vi "state-counter.vi"(10 "state-idx":u8) -> ()   [LabVIEW 2017]
uses:
  <vilib>/rvi/Emulation/niFpgaEmulationIsFPGAContextNoSignature.vi
  <vilib>/rvi/DataTransferAndStorage/Container/Common/niFpgaContainerGetUniqueNameForEmu.vi
  <vilib>/rvi/Memory/Memory_Emulation/niFpgaMemoryEmulationCacheClearOnFirstRun.vi
  <vilib>/rvi/Memory/Memory_Emulation/nirvimemoryEmulationManagerCache_MakeExclusive.vi
  <vilib>/rvi/Memory/Memory_Emulation/niFpgaMemoryEmulationValidateCache.vi
  <vilib>/rvi/Memory/Memory_Emulation/nirvimemoryEmulationManagerCache_InsertValue.vi
  <vilib>/Utility/error.llb/Clear Errors.vi
  <vilib>/rvi/Memory/Memory_Emulation/nirvimemoryEmulationManagerCache_ReleaseExclusive.vi
  <vilib>/rvi/Memory/Memory_Emulation/nirvimemoryEmulationManagerCache_GetValue.vi
  <vilib>/rvi/Memory/Memory_Emulation/nirvimemoryEmulationManagerCache_SetValue.vi
  <vilib>/rvi/Emulation/niFpgaProcessEmulError.vi
  <vilib>/rvi/Emulation/niFpgaSctlEmulationGetInTimedLoop.vi
  <vilib>/rvi/DataTransferAndStorage/Container/XNode/niFpgaContainer.xnode
  <vilib>/rvi/DataTransferAndStorage/Register/Emulation/niFpgaRegisterEmulation.vi
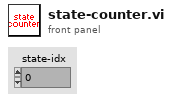
[diagram p1: front panel]
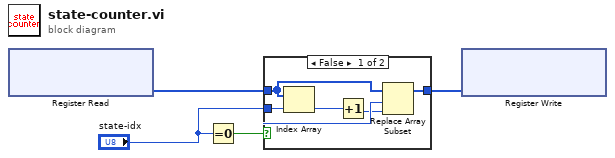
[diagram p0: block diagram]
diagram:
  n1 = xnode ("Register Read")() -> ("Data"=w4:u64[])  [unwired: 1 in, 1 out]
  n2 = Equal To 0?(x="state-idx") -> (x = 0?=w2:bool)
  n3 = case shown="False" w2 {
    tunnel: w4 -> [w7 w10]
    tunnel: [w8 w10] -> w3
    tunnel: "state-idx" -> [w6 _]
    frame False {
      n4 = Index Array(array=w7, index=w6) -> (element=w9:u64)
      n5 = Increment(x=w9) -> (x+1=w5:u64)
      n6 = Replace Array Subset(array=w7, new element=w5, index=w6) -> (w8:u64[])
    }
    frame True {
    }
  }
  n7 = xnode ("Register Write")("Data"=w3) -> ()  [unwired: 1 in, 1 out]
